vi "Get Additional data.vi"(11 "Additional Data":variant) -> (3 "Formated Additional data":string)   [LabVIEW 2023]
doc: "Converting data from Variant to defined data types and converting them to Formated string.\nPossible formats CAN message, LIN message, Number, Array of numbers, String"
uses:
  Communication/PLIN2023/PLIN2023/Controls/TLINRcvMsg.ctl
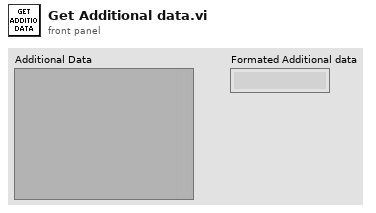
[diagram p1: front panel]
types:
  T1 = cluster{"ID":u32, "MSGTYPE":u8, "LEN":u8, "DATA[0]":u8, "DATA[1]":u8, "DATA[2]":u8, "DATA[3]":u8, "DATA[4]":u8, "DATA[5]":u8, "DATA[6]":u8, "DATA[7]":u8}
  T2 = typedef "PLinApi.lvlib/TLINRcvMsg.ctl" = cluster{"TLINMsgType":u8, "FrameID":u8, "Length":u8, "Direction":u8, "ChecksumType":u8, "Data [0]":u8, "Data [1]":u8, "Data [2]":u8, "Data [3]":u8, "Data [4]":u8, "Data [5]":u8, "Data [6]":u8, "Data [7]":u8, "Checksum":u8, "ErrorFlags":i32, "TimeStamp":u64, "hHw":u16}
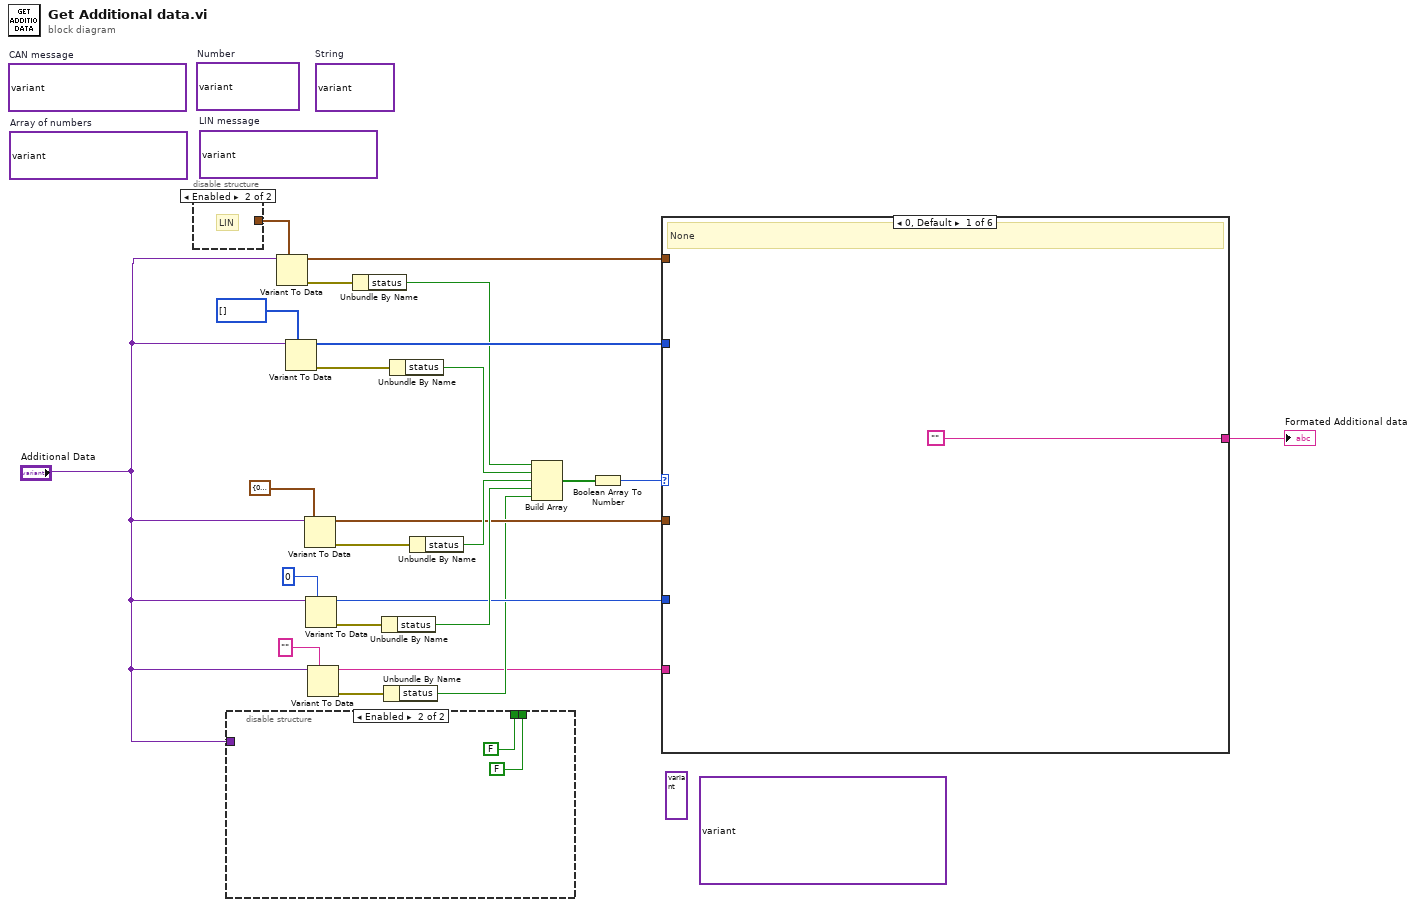
[diagram p0: block diagram]
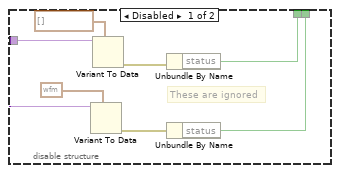
[diagram p2: hidden frame]
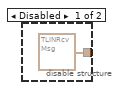
[diagram p3: hidden frame]
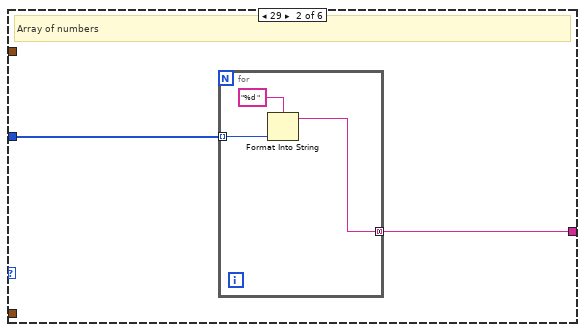
[diagram p4: hidden frame]
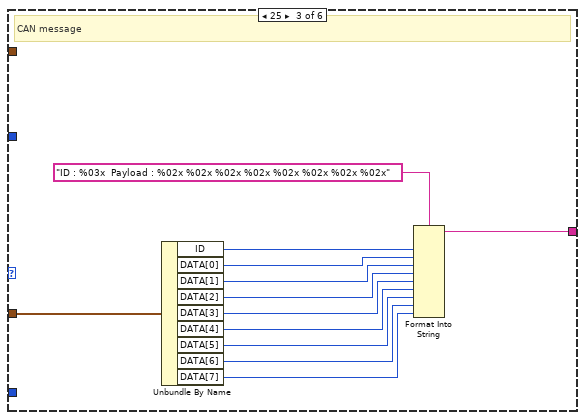
[diagram p5: hidden frame]
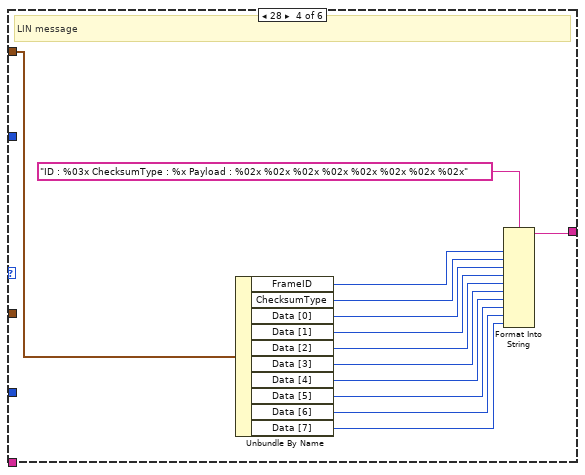
[diagram p6: hidden frame]
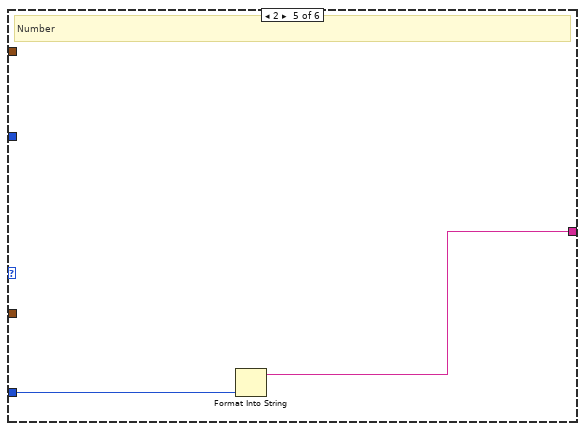
[diagram p7: hidden frame]
diagram:
  (unwired) variant(digitalwaveform {"t0"=timestamp(0 s since 1904-01-01), "dt"=0.0, "Y"={"transitions"=[], "data"=[]}}) ("variant 2")
  (unwired) variant(digitalwaveform[] []) ("variant")
  (unwired) variant  # String
  (unwired) variant  # LIN message
  (unwired) variant  # Number
  (unwired) variant  # Array of numbers
  (unwired) variant  # CAN message
  n1 = disable-structure shown="Enabled" {
    disable-tunnel: [T2 {"TLINMsgType"=0, "FrameID"=0, "Length"=0, "Direction"=0, "ChecksumType"=0, "Data [0]"=0, "Data [1]"=0, "Data [2]"=0, "Data [3]"=0, "Data [4]"=0, "Data [5]"=0, "Data [6]"=0, "Data [7]"=0, "Checksum"=0, "ErrorFlags"=0, "TimeStamp"=0, "hHw"=0} ("TLINRcvMsg") _] -> w10
    frame Disabled {
    }
    frame Enabled {
      # "LIN"
    }
  }
  n2 = disable-structure shown="Enabled" {
    disable-tunnel: [w28 FALSE ("status")] -> _
    disable-tunnel: [w27 FALSE ("status")] -> _
    disable-tunnel: "Additional Data" -> [w26 _]
    frame Disabled {
      # "These are ignored"
      n3 = Variant To Data(type=digitalwaveform {"t0"=timestamp(0 s since 1904-01-01), "dt"=0.0, "Y"={"transitions"=[], "data"=[]}} ("Digital Waveform Graph"), Variant=w26) -> (error out=w31:errorcluster)  [unwired: 1 in, 1 out]
      n4 = Variant To Data(type=digitalwaveform[] [] ("Digital Waveform Graph"), Variant=w26) -> (error out=w32:errorcluster)  [unwired: 1 in, 1 out]
      n5 = Unbundle By Name(w32) -> ("status"=w28:bool)
      n6 = Unbundle By Name(w31) -> ("status"=w27:bool)
    }
    frame Enabled {
    }
  }
  n7 = Variant To Data(type=w10, Variant="Additional Data") -> (data=w6:T2, error out=w8:errorcluster)  [unwired: 1 in]
  n8 = Variant To Data(type=i32[] [], Variant="Additional Data") -> (data=w12:i32[], error out=w21:errorcluster)  [unwired: 1 in]
  n9 = Variant To Data(type=T1 {"ID"=0, "MSGTYPE"=0, "LEN"=0, "DATA[0]"=0, "DATA[1]"=0, "DATA[2]"=0, "DATA[3]"=0, "DATA[4]"=0, "DATA[5]"=0, "DATA[6]"=0, "DATA[7]"=0} ("MessageBuffer out"), Variant="Additional Data") -> (data=w13:T1, error out=w7:errorcluster)  [unwired: 1 in]
  n10 = Variant To Data(type=0, Variant="Additional Data") -> (data=w14:i32, error out=w20:errorcluster)  [unwired: 1 in]
  n11 = Variant To Data(type="", Variant="Additional Data") -> (data=w2:string, error out=w5:errorcluster)  [unwired: 1 in]
  n12 = Unbundle By Name(w8) -> ("status"=w9:bool)
  n13 = Unbundle By Name(w20) -> ("status"=w17:bool)
  n14 = Unbundle By Name(w5) -> ("status"=w4:bool)
  n15 = Unbundle By Name(w21) -> ("status"=w19:bool)
  n16 = Unbundle By Name(w7) -> ("status"=w18:bool)
  n17 = Build Array(w9, w19, w18, w17, w4) -> (w16:bool[])
  n18 = Boolean Array To Number(Boolean array=w16) -> (number=w15:u32)
  n19 = case shown="0, Default" w15 {
    tunnel: w14 -> [_ _ _ _ w67 _]
    tunnel: w13 -> [_ _ w41 _ _ _]
    tunnel: w12 -> [_ w37 _ _ _ _]
    tunnel: ["" w36 w42 w54 w66 w68] -> w11
    tunnel: w6 -> [_ _ _ w53 _ _]
    tunnel: w2 -> [_ _ _ _ _ w68]
    frame 0, Default {
      # "None"
    }
    frame 29 {
      # "Array of numbers"
      n20 = for {
        tunnel: w37 -> [w40] mode=indexing
        tunnel: [w38] -> w36 mode=concatenating
        n21 = Format Into String(format string="%d ", w40) -> (resulting string=w38:string)  [unwired: 2 in, 1 out]
      }
    }
    frame 25 {
      # "CAN message"
      n22 = Unbundle By Name(w41) -> ("ID"=w51:u32, "DATA[0]"=w50:u8, "DATA[1]"=w49:u8, "DATA[2]"=w48:u8, "DATA[3]"=w47:u8, "DATA[4]"=w46:u8, "DATA[5]"=w45:u8, "DATA[6]"=w44:u8, "DATA[7]"=w43:u8)
      n23 = Format Into String(format string="ID : %03x  Payload : %02x %02x %02x %02x %02x %02x %02x %02x", w51, w50, w49, w48, w47, w46, w45, w44, w43) -> (resulting string=w42:string)  [unwired: 2 in, 1 out]
    }
    frame 28 {
      # "LIN message"
      n24 = Unbundle By Name(w53) -> ("FrameID"=w64:u8, "ChecksumType"=w63:u8, "Data [0]"=w62:u8, "Data [1]"=w61:u8, "Data [2]"=w60:u8, "Data [3]"=w59:u8, "Data [4]"=w58:u8, "Data [5]"=w57:u8, "Data [6]"=w56:u8, "Data [7]"=w55:u8)
      n25 = Format Into String(format string="ID : %03x ChecksumType : %x Payload : %02x %02x %02x %02x %02x %02x %02x %02x", w64, w63, w62, w61, w60, w59, w58, w57, w56, w55) -> (resulting string=w54:string)  [unwired: 2 in, 1 out]
    }
    frame 2 {
      # "Number"
      n26 = Format Into String(w67) -> (resulting string=w66:string)  [unwired: 3 in, 1 out]
    }
    frame 10 {
      # "String"
    }
  }
  "Formated Additional data" <- w11
